vi "LQR.vi"(6 "K":dbl[](array[numeric]) format="%#_13g", 8 "Steering angle in":dbl, 9 "Lean rate in":dbl, 10 "Lean angle in":dbl, 11 "Steering rate":dbl) -> (0 "Duty cycle":dbl, 1 "Cout":dbl, 2 "Direction":bool)   [LabVIEW 2016]
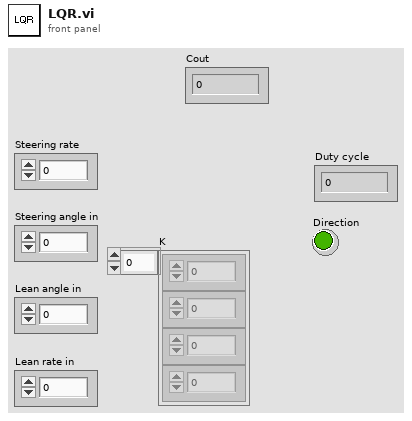
[diagram p1: front panel]
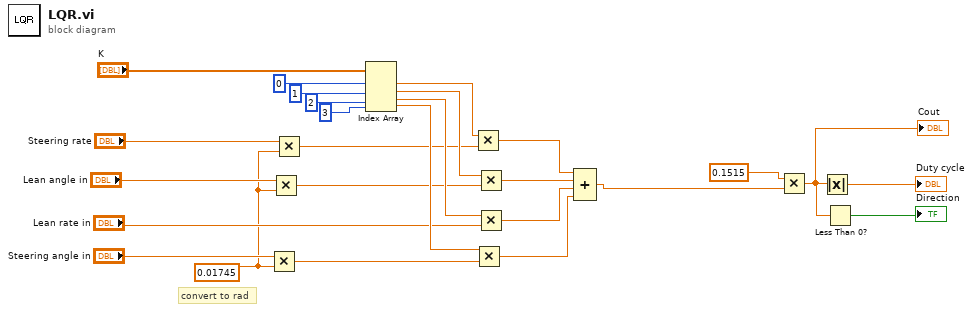
[diagram p0: block diagram]
diagram:
  w3 = 0.01745 ("x")
  # "convert to rad"
  n1 = Multiply(x="Steering angle in", y=w3) -> (x*y=w4:dbl)
  n2 = Multiply(x="Lean angle in", y=w3) -> (x*y=w6:dbl)
  n3 = Multiply(x="Steering rate", y=w3) -> (x*y=w7:dbl)
  n4 = Index Array(array="K", index #1=0 ("index"), index #2=1 ("index"), index #3=2 ("index"), index #4=3 ("index")) -> (element #1=w15:dbl, element #2=w14:dbl, element #3=w13:dbl, element #4=w16:dbl)
  n5 = Multiply(x=w15, y=w7) -> (x*y=w12:dbl)
  n6 = Multiply(x=w16, y=w4) -> (x*y=w9:dbl)
  n7 = Multiply(x=w14, y=w6) -> (x*y=w11:dbl)
  n8 = Multiply(x=w13, y="Lean rate in") -> (x*y=w10:dbl)
  n9 = Compound Arithmetic op=ADD(w12, w11, w10, w9) -> (w2:dbl)
  n10 = Multiply(x=0.1515, y=w2) -> (x*y=w1:dbl)
  "Cout" <- w1
  n11 = Absolute Value(x=w1) -> (abs(x)=→"Duty cycle":dbl)
  n12 = Less Than 0?(x=w1) -> (x < 0?=→"Direction":bool)
